vi "request.Has ID.vi"(8 "error in (no error)":errorcluster, 11 "Request in":refnum<class "Request.lvclass">) -> (0 "error out":errorcluster, 2 "has id?":bool, 3 "Request out":refnum<class "Request.lvclass">)   [LabVIEW 2020, in "JSON-RPC Lib.lvlib" / "Request.lvclass"]
uses:
  Request.lvclass
  Request.lvclass/Request.ctl
  id/id.lvclass
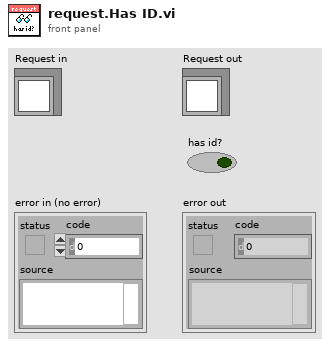
[diagram p1: front panel]
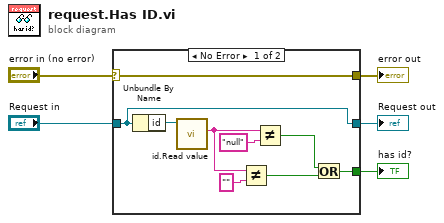
[diagram p0: block diagram]
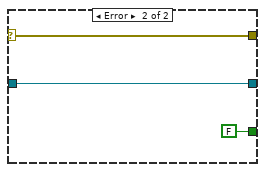
[diagram p2: hidden frame]
diagram:
  n1 = case shown="No Error" "error in (no error)" {
    selector: "error in (no error)" -> [w14 w16]
    tunnel: [w14 w16] -> w4
    tunnel: [w13 w17] -> w2
    tunnel: "Request in" -> [w13 w17]
    tunnel: [w8 FALSE] -> w1
    frame No Error {
      n2 = Unbundle By Name(w13) -> ("id"=w7:refnum<class "id.lvclass">)
      n3 = call "id.Read value.vi"("id in"=w7) -> ("value"=w6:string)  [unwired: 8 in, 2 out]
      n4 = Not Equal?(x=w6, y="") -> (x != y?=w12:bool)
      n5 = Not Equal?(x=w6, y="null") -> (x != y?=w11:bool)
      n6 = Or(x=w11, y=w12) -> (x .or. y?=w8:bool)
    }
    frame Error {
    }
  }
  "error out" <- w4
  "Request out" <- w2
  "has id?" <- w1
